vi "Library Line at Offset.vi"(7 "multi-line string":string, 11 "offset in string":i32) -> (8 "line number":i32)   [LabVIEW 2012]
doc: "Determines the linenumber (counting from 1) at an offset in a multi-line string."
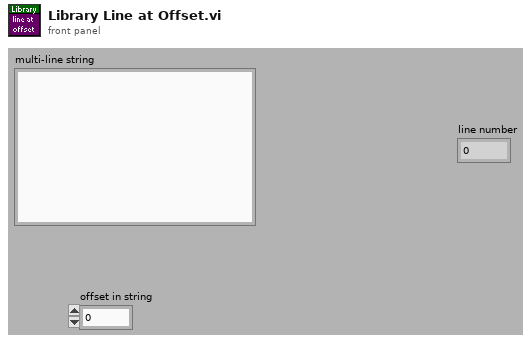
[diagram p1: front panel]
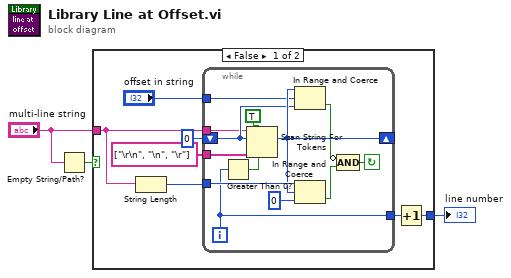
[diagram p0: block diagram]
diagram:
  n1 = Empty String/Path?(string/path="multi-line string") -> (empty?=w2:bool)
  n2 = case shown="False" w2 {
    tunnel: "multi-line string" -> [w4 _]
    tunnel: [w5 _] -> w1
    frame False {
      n3 = String Length(string=w4) -> (length=w8:i32)
      n4 = while {
        tunnel: string[] ["\r\n", "\n", "\r"] ("delimiters (\\s,\\t,\\r,\\n)") -> [w23]
        shift-right: [w17] -> _
        shift-left: 0 ("offset past token") -> [w16]
        tunnel: w8 -> [w21]
        tunnel: [w18] -> w7
        tunnel: "offset in string" -> [w15]
        tunnel: w4 -> [w11]
        i -> [w18]
        stop <- w12 continue-if-true
        n5 = Greater Than 0?(x=w18) -> (x > 0?=w20:bool)
        n6 = Scan String For Tokens(4:w20, 5:TRUE ("allow empty tokens? (F)"), 6:w23, 8:w16, 9:w11) -> (2:w17:i32)  [unwired: 1 in, 3 out]
        n7 = In Range and Coerce(upper limit=w17, x=w15, lower limit=w16) -> (In Range?=w13:bool)  [unwired: 1 out]
        n8 = In Range and Coerce(upper limit=w21, x=w17, lower limit=0) -> (In Range?=w14:bool)  [unwired: 1 out]
        n9 = Compound Arithmetic op=AND(invert w13, w14) -> (w12:bool)
      }
      n10 = Increment(x=w7) -> (x+1=w5:i32)
    }
    frame True {
    }
  }
  "line number" <- w1
